vi "Render Window Redraw.vi"(6 "Control Ref Queue":T1, 8 "error in (no error)":errorcluster) -> (0 "error out":errorcluster)   [LabVIEW 2020, in "3D Plot.lvclass"]
uses:
  3D Plot.lvclass
  3DMathPlot Ctrl Act Queue.ctl
  3DMathPlot Ctrl Act Cluster.ctl
  3DMathPlot State Class.ctl
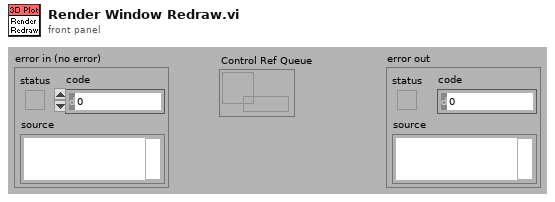
[diagram p1: front panel]
types:
  T1 = typedef "3DMathPlot Ctrl Act Queue.ctl" = refnum<queue>
  T2 = typedef "3DMathPlot Ctrl Act Cluster.ctl" = cluster{"3D Picture Control":refnum<vi>, "Render Window Refnum":refnum<vi>, "XY Graph":refnum<vi>, "Intensity Graph":refnum<vi>, "Color Legend Palette":refnum<vi>, "Projection Palette":refnum<vi>, "XControl  Ref":refnum<vi>, "Facade Ref":refnum<vi>, "Export Image Ref":refnum<vi>, "Clear Data Flag":bool, "Display State Change Class":T3}
  T3 = typedef "3DMathPlot State Class.ctl" = enum16{"Update All Objects (Undo)", "Update Light Object Only", "Update Axis Object Only", "Update Plot Object Only", "Update Cursor Object Only", "Update Axis Plot Cursor Objects", "No Update"}
  T4 = enum16{"Open", "Minimized", "Maximized", "Hidden"}
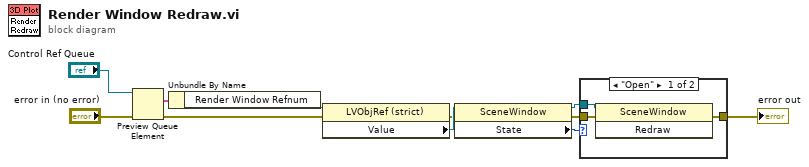
[diagram p0: block diagram]
diagram:
  n1 = Preview Queue Element(queue="Control Ref Queue", error in (no error)="error in (no error)") -> (element=w7:T2, error out=w1:errorcluster)  [unwired: 3 out]
  n2 = Unbundle By Name(w7) -> ("Render Window Refnum"=w8:refnum<vi>)
  n3 = property class="LVObjRef (strict)"(reference=w8, error in=w1) -> (error out=w2:errorcluster, "Value"=w3:refnum<vi>)  [unwired: 1 out]
  n4 = property class="SceneWindow"(reference=w3, error in=w2) -> (reference out=w4:refnum<vi>, error out=w6:errorcluster, "State"=w5:T4)
  n5 = case shown="\"Open\"" w5 {
    tunnel: w4 -> [w14 _]
    tunnel: w6 -> [w13 w15]
    tunnel: [w12 w15] -> w11
    frame "Open" {
      n6 = invoke class="SceneWindow" method="Redraw"(reference=w14, error in=w13) -> (error out=w12:errorcluster)  [unwired: 1 in, 2 out]
    }
    frame Default {
    }
  }
  "error out" <- w11
